vi "Number to String.vi"(11 "DecimaL NU\nmber":i32) -> (3 "Decimal String":string)   [LabVIEW 2021]
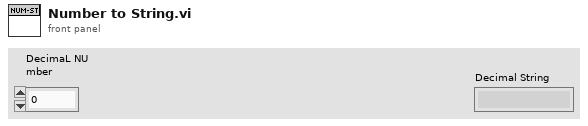
[diagram p1: front panel]
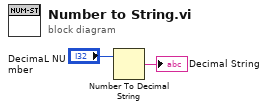
[diagram p0: block diagram]
diagram:
  n1 = Number To Decimal String(number="DecimaL NU\nmber") -> (decimal integer string=→"Decimal String":string)  [unwired: 1 in]
